vi "calculate gradient output.vi"(7 "enabled":bool, 10 "t0":u32, 11 "gradient parameters":T1={"temporal ramp type"=enum."Sine", "period(s)"=120.0, "high limit"=100.0, "low limit"=0.0, "duty cycle (sq wave)"=50.0, "phase shift (deg)"=0.0, "value to output when disabled"=0.0} {"value to output when disabled" max=100.0; "low limit" min=0.0 max=1.0 format="%#_6p"; "high limit" max=100.0}) -> (3 "value out":dbl)   [LabVIEW 2021]
uses:
  <vilib>/ptbypt/NI_PtbyPt.lvlib
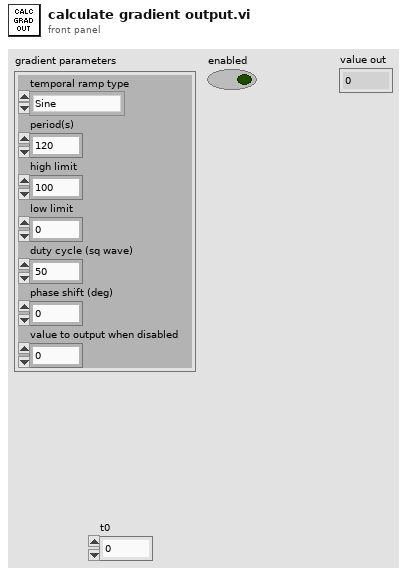
[diagram p1: front panel]
types:
  T1 = cluster{"temporal ramp type":enum16{"Sine", "Triangle", "Sawtooth", "Square", "Exponential"}, "period(s)":dbl, "high limit":dbl, "low limit":dbl, "duty cycle (sq wave)":dbl, "phase shift (deg)":dbl, "value to output when disabled":dbl}
  T2 = enum16{"Sine", "Triangle", "Sawtooth", "Square", "Exponential"}
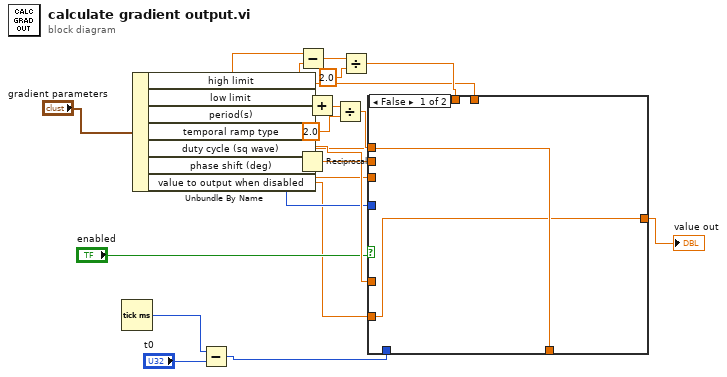
[diagram p0: block diagram]
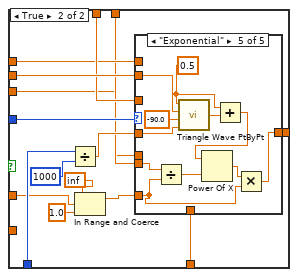
[diagram p2: hidden frame]
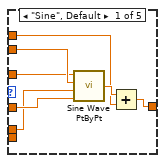
[diagram p3: hidden frame]
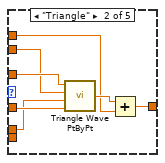
[diagram p4: hidden frame]
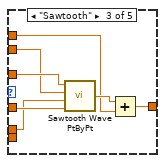
[diagram p5: hidden frame]
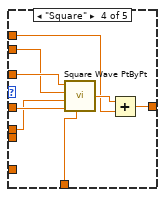
[diagram p6: hidden frame]
diagram:
  n1 = Tick Count (ms)() -> (millisecond timer value=w2:u32)
  n2 = Unbundle By Name("gradient parameters") -> ("high limit"=w17:dbl, "low limit"=w20:dbl, "period(s)"=w14:dbl, "temporal ramp type"=w19:T2, "duty cycle (sq wave)"=w8:dbl, "phase shift (deg)"=w5:dbl, "value to output when disabled"=w1:dbl)
  n3 = Subtract(x=w2, y="t0") -> (x-y=w3:u32)
  n4 = Reciprocal(x=w14) -> (1/x=w10:dbl)
  n5 = Subtract(x=w17, y=w20) -> (x-y=w4:dbl)
  n6 = Add(x=w17, y=w20) -> (x+y=w11:dbl)
  n7 = Divide(x=w11, y=2.0) -> (x/y=w13:dbl)
  n8 = Divide(x=w4, y=2.0) -> (x/y=w18:dbl)
  n9 = case shown="False" "enabled" {
    tunnel: w3 -> [_ w36]
    tunnel: w10 -> [_ w33]
    tunnel: w18 -> [_ w32]
    tunnel: w13 -> [_ w31]
    tunnel: [w21 w30] -> w9
    tunnel: w19 -> [_ w29]
    tunnel: w20 -> [_ w26]
    tunnel: w17 -> [_ w28]
    tunnel: w8 -> [_ w24]
    tunnel: w5 -> [_ w22]
    tunnel: w1 -> [w21 _]
    frame False {
    }
    frame True {
      n10 = Divide(x=w36, y=u32 1000) -> (x/y=w35:dbl)
      n11 = In Range and Coerce(upper limit=inf, x=w26, lower limit=1.0) -> (coerced(x)=w27:dbl)  [unwired: 1 out]
      n12 = case shown="\"Exponential\"" w29 {
        tunnel: w35 -> [w43 w46 w53 w61 w76]
        tunnel: w33 -> [w42 w48 w55 w63 w74]
        tunnel: w32 -> [w41 w49 w56 w64 _]
        tunnel: w31 -> [w39 w47 w54 w62 _]
        tunnel: [w38 w45 w52 w60 w66] -> w30
        tunnel: w27 -> [_ _ _ _ w67]
        tunnel: w28 -> [_ _ _ _ w71]
        tunnel: w24 -> [_ _ _ w59 _]
        tunnel: w22 -> [w37 w44 w51 w58 _]
        frame "Sine", Default {
          n13 = call <vilib>:"Sine Wave PtByPt.vi"("time"=w43, "phase"=w37, "frequency"=w42, "amplitude"=w41) -> ("sine wave"=w40:dbl)
          n14 = Add(x=w40, y=w39) -> (x+y=w38:dbl)
        }
        frame "Triangle" {
          n15 = call <vilib>:"Triangle Wave PtByPt.vi"("time"=w46, "phase"=w44, "frequency"=w48, "amplitude"=w49) -> ("triangle wave"=w50:dbl)
          n16 = Add(x=w50, y=w47) -> (x+y=w45:dbl)
        }
        frame "Sawtooth" {
          n17 = call <vilib>:"Sawtooth Wave PtByPt.vi"("time"=w53, "phase"=w51, "frequency"=w55, "amplitude"=w56) -> ("sawtooth wave"=w57:dbl)
          n18 = Add(x=w57, y=w54) -> (x+y=w52:dbl)
        }
        frame "Square" {
          n19 = call <vilib>:"Square Wave PtByPt.vi"("amplitude"=w64, "frequency"=w63, "phase"=w58, "time"=w61, "duty cycle (%)"=w59) -> ("square wave"=w65:dbl)
          n20 = Add(x=w65, y=w62) -> (x+y=w60:dbl)
        }
        frame "Exponential" {
          w72 = 0.5 ("amplitude")
          n21 = Divide(x=w71, y=w67) -> (x/y=w70:dbl)
          n22 = call <vilib>:"Triangle Wave PtByPt.vi"("time"=w76, "phase"=-90.0, "frequency"=w74, "amplitude"=w72) -> ("triangle wave"=w73:dbl)
          n23 = Add(x=w72, y=w73) -> (x+y=w69:dbl)
          n24 = Power Of X(1:w70, 2:w69) -> (0:w68:dbl)
          n25 = Multiply(x=w68, y=w67) -> (x*y=w66:dbl)
        }
      }
    }
  }
  "value out" <- w9
